vi "Flatten Test Executive.vi"(4 "New GUIDs":bool, 6 "Persistence in":refnum<class "IPersist.lvclass">, 7 "Root ID":string, 8 "error in (no error)":errorcluster, 11 "Test Executive Ref":refnum<data-value>) -> (0 "error out":errorcluster, 2 "Flattened Test Executive":string, 3 "Test Executive Ref out":refnum<data-value>)   [LabVIEW 2019, in "Test Executive.lvlib" / "TestExecutive Ref.lvclass"]
uses:
  <vilib>/gpm_packages/@cs/test-executive/Source/Test Executive/TestExecutive Ref/TestExecutive Ref.lvclass
  <vilib>/gpm_packages/@cs/test-executive/Source/Test Executive/ITestExecutive/ITest Executive.lvclass
  <vilib>/gpm_packages/@cs/persistence/source/IPersist/IPersist.lvclass
  <vilib>/gpm_packages/@cs/linked-list/Source/String Manipulation/String Manipulation.lvlib
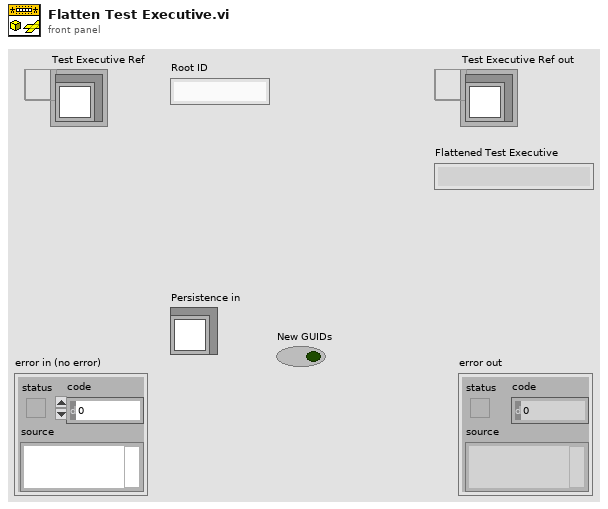
[diagram p1: front panel]
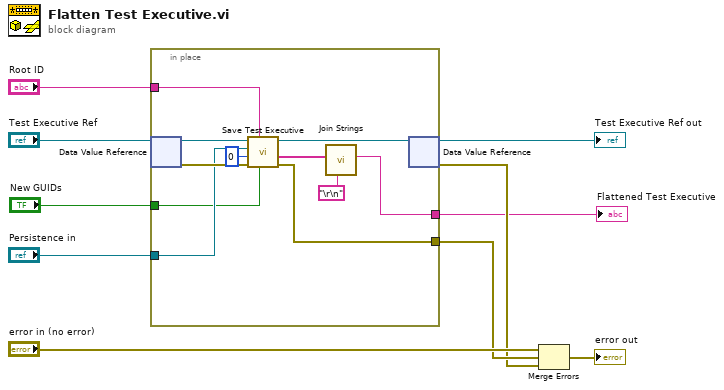
[diagram p0: block diagram]
diagram:
  n1 = in-place {
    in-place-border: "Root ID" -> [w17]
    in-place-border: [w18] -> w6
    in-place-border: "Persistence in" -> [w16]
    in-place-border: [w13] -> w2
    in-place-border: "New GUIDs" -> [w11]
    n2 = in-place-dvr #1("Test Executive Ref") -> (w21:refnum<class "ITest Executive.lvclass">, w20:errorcluster)
    n3 = call-dynamic "Save Test Executive.vi"("New GUIDs"=w11, "Root ID"=w17, "error in (no error)"=w20, "Indent"=0, "Persistence in"=w16, "ITest Executive in"=w21) -> ("error out"=w18:errorcluster, "Flattened Test Executive"=w14:string[], "ITest Executive out"=w19:refnum<class "ITest Executive.lvclass">)  [unwired: 2 in, 1 out]
    n4 = call <vilib>:"Join Strings.vi"("Separator (,)"="\r\n", "Strings In"=w14) -> ("String"=w13:string)  [unwired: 9 in]
    n5 = in-place-dvr #1(w19) -> (→"Test Executive Ref out":refnum<data-value>, w5:errorcluster)
  }
  "Flattened Test Executive" <- w2
  n6 = Merge Errors("error in (no error)", w6, w5) -> (→"error out":errorcluster)
